vi "CalculateMcsaSpeed[m].vi"(6 "Calculation Cache In":T3 {"speed initial conditions"."zoom FFT settings"."FFT settings"."window" items=["Rectangle"=0, "Hanning"=1, "Hamming"=2, "Blackman-Harris"=3, "Exact Blackman"=4, "Blackman"=5, "Flat Top"=6, "4 Term B-Harris "=7, "7 Term B-Harris"=8, "Low Sidelobe"=9, "Blackman Nuttall"=11, "Triangle"=30, "Bartlett-Hanning"=31, "Bohman"=32, "Parzen"=33, "Welch"=34, "Kaiser"=60, "Dolph-Chebyshev"=61, "Gaussian"=62]; "spectrum initial conditions"."zoom FFT settings"."FFT settings"."window" items=["Rectangle"=0, "Hanning"=1, "Hamming"=2, "Blackman-Harris"=3, "Exact Blackman"=4, "Blackman"=5, "Flat Top"=6, "4 Term B-Harris "=7, "7 Term B-Harris"=8, "Low Sidelobe"=9, "Blackman Nuttall"=11, "Triangle"=30, "Bartlett-Hanning"=31, "Bohman"=32, "Parzen"=33, "Welch"=34, "Kaiser"=60, "Dolph-Chebyshev"=61, "Gaussian"=62]}, 7 "nameplate information":T2, 8 "error in (no error)":errorcluster, 9 "Map":T1, 10 "current waveform":waveform(dbl)[](array[waveform]), 11 "voltage waveform":waveform(dbl)[](array[waveform])) -> (0 "error out":errorcluster, 3 "speed [RPM]":dbl, 4 "Calculation Cache Out":T3 {"speed initial conditions"."zoom FFT settings"."FFT settings"."window" items=["Rectangle"=0, "Hanning"=1, "Hamming"=2, "Blackman-Harris"=3, "Exact Blackman"=4, "Blackman"=5, "Flat Top"=6, "4 Term B-Harris "=7, "7 Term B-Harris"=8, "Low Sidelobe"=9, "Blackman Nuttall"=11, "Triangle"=30, "Bartlett-Hanning"=31, "Bohman"=32, "Parzen"=33, "Welch"=34, "Kaiser"=60, "Dolph-Chebyshev"=61, "Gaussian"=62]; "spectrum initial conditions"."zoom FFT settings"."FFT settings"."window" items=["Rectangle"=0, "Hanning"=1, "Hamming"=2, "Blackman-Harris"=3, "Exact Blackman"=4, "Blackman"=5, "Flat Top"=6, "4 Term B-Harris "=7, "7 Term B-Harris"=8, "Low Sidelobe"=9, "Blackman Nuttall"=11, "Triangle"=30, "Bartlett-Hanning"=31, "Bohman"=32, "Parzen"=33, "Welch"=34, "Kaiser"=60, "Dolph-Chebyshev"=61, "Gaussian"=62]})   [LabVIEW 2017, in "McsaAnalysisFunctions.lvlib"]
uses:
  <vilib>/addons/InsightCM/Utilities/Analysis/MCSA/McsaAnalysisFunctions.lvlib
  <vilib>/addons/InsightCM/Utilities/Analysis/MCSA/controls/McsaCalculationCache.ctl
  <vilib>/addons/Electrical Power/Motor Monitoring/subVIs/ep_Initial Conditions for MCSA Spectra.ctl
  <vilib>/addons/Electrical Power/Motor Monitoring/subVIs/ep_Demodulation Algorithm.ctl
  <vilib>/addons/Electrical Power/Motor Monitoring/subVIs/ep_Zoom FFT Settings.ctl
  <vilib>/addons/Electrical Power/Motor Monitoring/subVIs/ep_Initial Conditions for Speed Estimation.ctl
  <vilib>/addons/PointValueMap/controls/PointMap.ctl
  <vilib>/addons/Electrical Power/Motor Monitoring/subVIs/ep_Spectra Settings.ctl
  <vilib>/addons/Electrical Power/Motor Monitoring/MCSA Spectra (1 Motor with IC).vi
  <vilib>/addons/Electrical Power/Motor Monitoring/NI_EP_Motor Monitoring.lvlib
  <vilib>/addons/PointValueMap/PointValueMap.lvlib
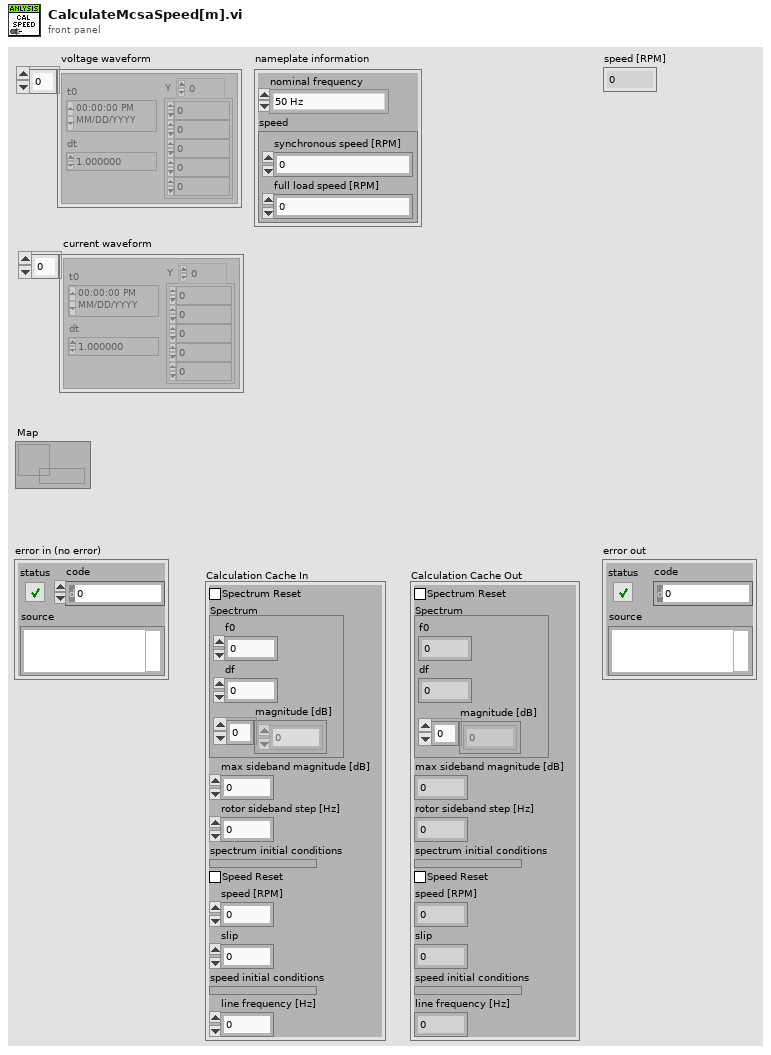
[diagram p1: front panel]
types:
  T1 = typedef "PointValueMap.lvlib/PointMap.ctl" = refnum<data-value>
  T2 = cluster{"nominal frequency":enum16{"50 Hz", "60 Hz"}, "speed":cluster{"synchronous speed [RPM]":dbl, "full load speed [RPM]":dbl}}
  T3 = typedef "McsaAnalysisFunctions.lvlib/McsaCalculationCache.ctl" = cluster{"Spectrum Reset":bool, "Spectrum":cluster{"f0":dbl, "df":dbl, "magnitude [dB]":dbl[]}, "max sideband magnitude [dB]":dbl, "rotor sideband step [Hz]":dbl, "spectrum initial conditions":T4, "Speed Reset":bool, "speed [RPM]":dbl, "slip":dbl, "speed initial conditions":T7, "line frequency [Hz]":dbl}
  T4 = typedef "NI_EP_Motor Monitoring.lvlib/ep_Initial Conditions for MCSA Spectra.ctl" = cluster{"hilbert state":cluster{"delay conditions":dbl[], "filter conditions":dbl[]}, "zoom FFT state":cluster{"phase state":dbl, "zoom FFT state":cluster{"zoom settings state":cluster{"zoom":i32, "stop band attenuation":enum16{"84 dB", "96 dB", "120 dB"}, "alias protect in final transition":bool, "oversampling ratio":dbl}, "SML Decimation Filter (complex input) state":cluster{"decimation settings state":cluster{"M":i32, "stop band attenuation":enum16{"84 dB", "96 dB", "120 dB"}, "alias protect in transition band":bool, "oversampling ratio":dbl}, "counter for garbage samples state":i32, "sml_Parameter Setting for Zoom Factor state":cluster{"filter length * interpolation state":i32, "interpolation state":i32, "comb filter order state":i32, "CFIR par state":cluster{"h":dbl[], "M":i32, "N":i32}, "LFIR par state":cluster{"h":dbl[], "M":i32, "N":i32}, "CIC Stages state":i32}, "aal_CIC (complex input) state":cluster{"aal_cascaded moving average (complex input) state":cluster{"states":cdb[], "circular buffers state":cdb[][], "circular buffer counter state":i32}, "aal_moving average with decimation by order (complex input) state":cluster{"residue result state":cdb, "processed data counter state":i32}}, "sml_Cascaded Decimation Filter (complex input) CFIR state":cluster{"unprocessed data state":cdb[], "final conditions state":cdb[][], "sml_M-1 Decimator with IC (complex input) state":cluster{"coefficients in reverse order state":dbl[], "max index for coefficients state":i32}}, "sml_Cascaded Decimation Filter (complex input) LFIR state":cluster{"unprocessed data state":cdb[], "final conditions state":cdb[][], "sml_M-1 Decimator with IC (complex input) state":cluster{"coefficients in reverse order state":dbl[], "max index for coefficients state":i32}}}, "ma_SML Data Packing (complex input) state":cluster{"array getting packed state":cdb[], "last array processed state":cdb[], "index state":i32, "packing parameters state":cluster{i32, "size":i32}}}, "FFT{X} [Vrms]":cdb[]}, "IIR filter state":cluster{"filter state":dbl[]}, "demodulation settings":cluster{"enable? (F)":bool, "algorithm":T5}, "highpass IIR Filter":cluster{"filter structure":enum32{"IIR 2nd Order", "IIR 4th Order"}, "Reverse Coefficients":dbl[], "Forward Coefficients":dbl[]}, "Hilbert FIR filter":cluster{"coefficients":dbl[], "delay":i32}, "zoom FFT settings":T6}
  T5 = typedef "NI_EP_Motor Monitoring.lvlib/ep_Demodulation Algorithm.ctl" = enum16{"1-phase signal", "3-phase signals"}
  T6 = typedef "NI_EP_Motor Monitoring.lvlib/ep_Zoom FFT Settings.ctl" = cluster{"FFT settings":cluster{"window":u16, "Window Size":i32, "FFT Size":i32, "%overlap":dbl}, "zoom settings":cluster{"zoom":i32, "stop band attenuation":enum16{"84 dB", "96 dB", "120 dB"}, "alias protect in final transition":bool, "oversampling ratio":dbl}, "other settings":cluster{"fmod":dbl, "f0":dbl, "df":dbl, "oidx":i32, "olen":i32}, "iterations":i32, "max block size":i32, "fs":dbl}
  T7 = typedef "NI_EP_Motor Monitoring.lvlib/ep_Initial Conditions for Speed Estimation.ctl" = cluster{"SVAF state":cluster{"space vector amplitude":dbl, "hilbert state":cluster{"delay conditions":dbl[], "filter conditions":dbl[]}}, "zoom FFT state":cluster{"phase state":dbl, "zoom FFT state":cluster{"zoom settings state":cluster{"zoom":i32, "stop band attenuation":enum16{"84 dB", "96 dB", "120 dB"}, "alias protect in final transition":bool, "oversampling ratio":dbl}, "SML Decimation Filter (complex input) state":cluster{"decimation settings state":cluster{"M":i32, "stop band attenuation":enum16{"84 dB", "96 dB", "120 dB"}, "alias protect in transition band":bool, "oversampling ratio":dbl}, "counter for garbage samples state":i32, "sml_Parameter Setting for Zoom Factor state":cluster{"filter length * interpolation state":i32, "interpolation state":i32, "comb filter order state":i32, "CFIR par state":cluster{"h":dbl[], "M":i32, "N":i32}, "LFIR par state":cluster{"h":dbl[], "M":i32, "N":i32}, "CIC Stages state":i32}, "aal_CIC (complex input) state":cluster{"aal_cascaded moving average (complex input) state":cluster{"states":cdb[], "circular buffers state":cdb[][], "circular buffer counter state":i32}, "aal_moving average with decimation by order (complex input) state":cluster{"residue result state":cdb, "processed data counter state":i32}}, "sml_Cascaded Decimation Filter (complex input) CFIR state":cluster{"unprocessed data state":cdb[], "final conditions state":cdb[][], "sml_M-1 Decimator with IC (complex input) state":cluster{"coefficients in reverse order state":dbl[], "max index for coefficients state":i32}}, "sml_Cascaded Decimation Filter (complex input) LFIR state":cluster{"unprocessed data state":cdb[], "final conditions state":cdb[][], "sml_M-1 Decimator with IC (complex input) state":cluster{"coefficients in reverse order state":dbl[], "max index for coefficients state":i32}}}, "ma_SML Data Packing (complex input) state":cluster{"array getting packed state":cdb[], "last array processed state":cdb[], "index state":i32, "packing parameters state":cluster{i32, "size":i32}}}, "FFT{X} [Vrms]":cdb[]}, "speed state":cluster{"speed [RPM]":dbl, "slip":dbl}, "speed estimation settings":cluster{"% overlap":dbl, "algorithm":T5}, "filter information":cluster{"coefficients":dbl[], "order":i32}, "zoom FFT settings":T6, "last valid window":i32, "fund. frequency for averager":dbl[]}
  T8 = typedef "NI_EP_Motor Monitoring.lvlib/ep_Spectra Settings.ctl" = cluster{"number of lines":i32, "% overlap":dbl, "maximum frequency [Hz]":dbl}
  T9 = cluster{"f0":dbl, "df":dbl, "magnitude [dB]":dbl[]}
  T10 = cluster{"spectrum":cluster{"f0":dbl, "df":dbl, "magnitude [dB]":dbl[]}, "demodulated?":bool}
  T11 = cluster{"sideband frequency [Hz]":dbl[], "sideband magnitude [dB]":dbl[]}
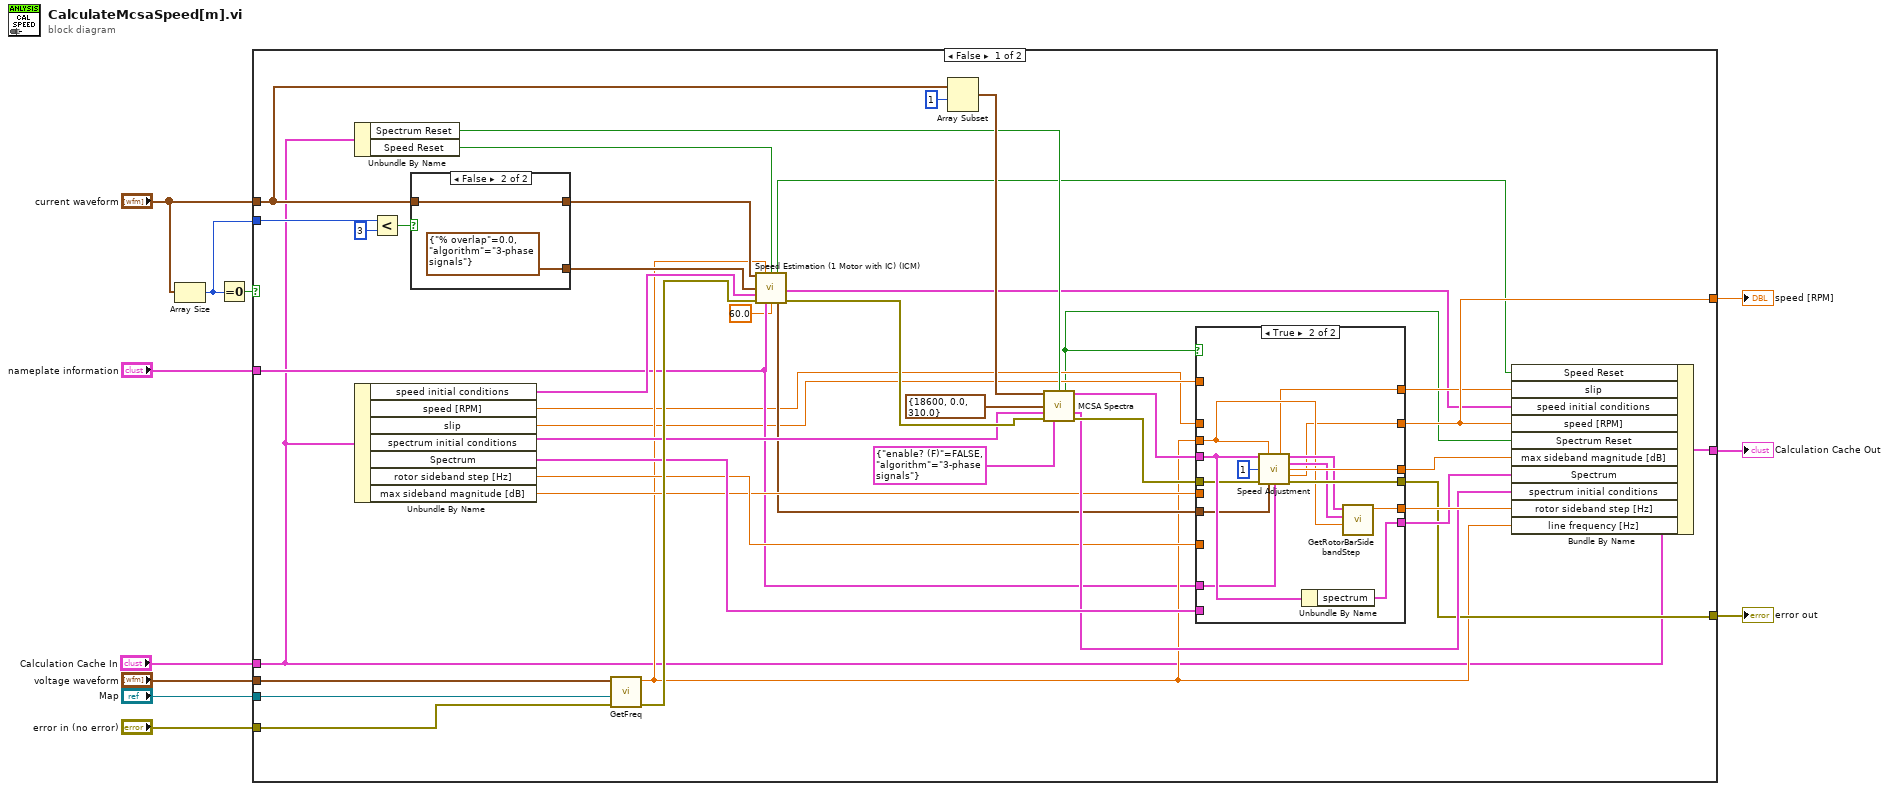
[diagram p0: block diagram]
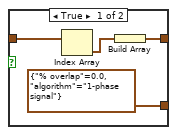
[diagram p3: hidden frame]
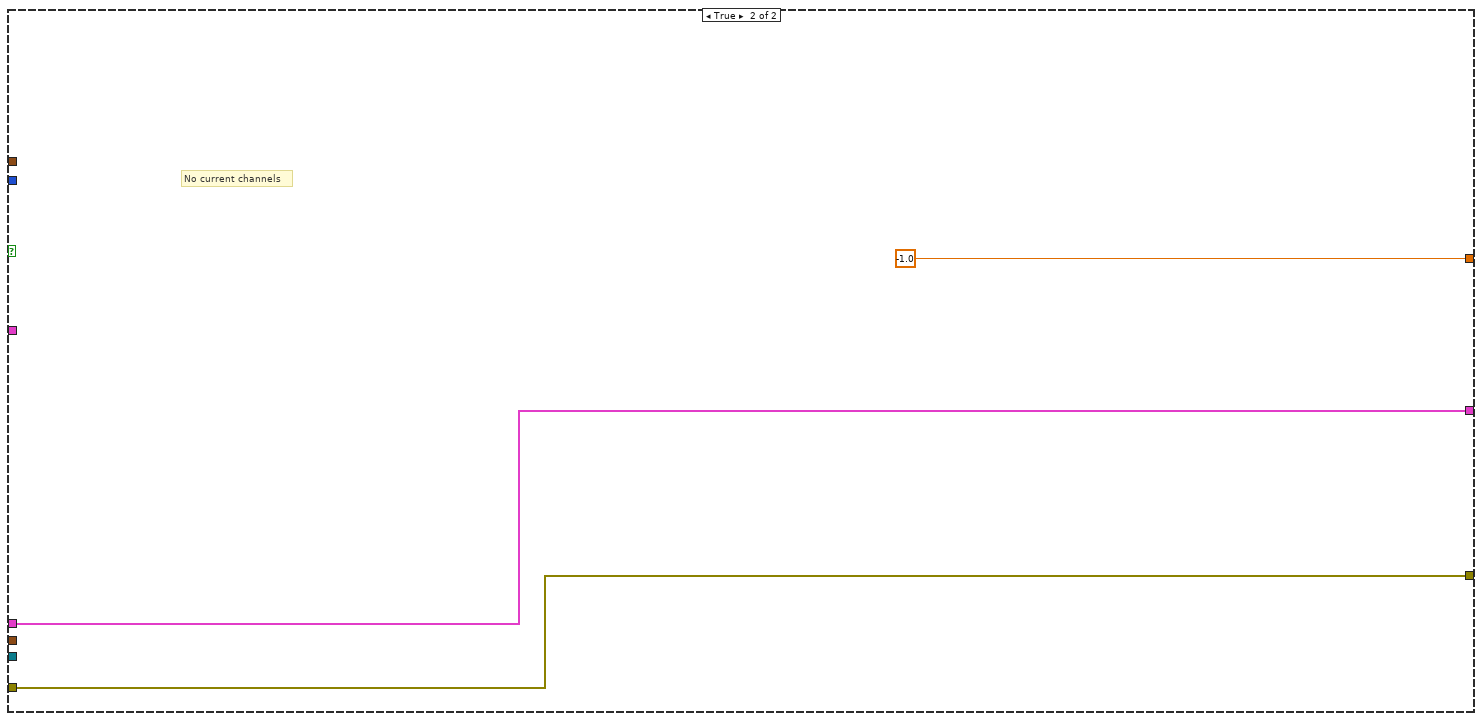
[diagram p4: hidden frame]
diagram:
  n1 = Array Size(array="current waveform") -> (size(s)=w1:i32)
  n2 = Equal To 0?(x=w1) -> (x = 0?=w2:bool)
  n3 = case shown="False" w2 {
    tunnel: "current waveform" -> [w24 _]
    tunnel: [w26 w81] -> w11
    tunnel: [w21 -1.0 ("speed [RPM]")] -> w10
    tunnel: "nameplate information" -> [w20 _]
    tunnel: [w27 w80] -> w8
    tunnel: "error in (no error)" -> [w47 w80]
    tunnel: "Calculation Cache In" -> [w16 w81]
    tunnel: "Map" -> [w46 _]
    tunnel: "voltage waveform" -> [w45 _]
    tunnel: w1 -> [w44 _]
    frame False {
      n4 = Unbundle By Name(w16) -> ("Spectrum Reset"=w36:bool, "Speed Reset"=w51:bool)
      n5 = Unbundle By Name(w16) -> ("speed initial conditions"=w49:T7, "speed [RPM]"=w13:dbl, "slip"=w17:dbl, "spectrum initial conditions"=w37:T4, "Spectrum"=w33:T9, "rotor sideband step [Hz]"=w29:dbl, "max sideband magnitude [dB]"=w28:dbl)
      n6 = Less?(x=w44, y=3) -> (x < y?=w52:bool)
      n7 = case shown="False" w52 {
        tunnel: w24 -> [w77 w79]
        tunnel: [w75 w79] -> w43
        tunnel: [cluster{"% overlap":dbl, "algorithm":T5} {"% overlap"=0.0, "algorithm"=enum."1-phase signal"} ("speed estimation settings") cluster{"% overlap":dbl, "algorithm":T5} {"% overlap"=0.0, "algorithm"=enum."3-phase signals"} ("speed estimation settings")] -> w50
        frame True {
          n8 = Index Array(array=w77) -> (element=w76:waveform(dbl))  [unwired: 1 in]
          n9 = Build Array(w76) -> (w75:waveform(dbl)[])
        }
        frame False {
        }
      }
      n10 = call <vilib>:"GetFreq.vi"("error in (no error)"=w47, "Map"=w46, "waveforms"=w45) -> ("error out"=w48:errorcluster, "frequency"=w23:dbl)  [unwired: 7 in]
      n11 = call <vilib>:"Speed Estimation (1 Motor with IC) (ICM).vi"("waveforms"=w43, "fundamental frequency [Hz]"=w23, "reset? (F)"=w51, "speed estimation settings"=w50, "initial conditions"=w49, "error in (no error)"=w48, "nameplate information"=w20, "window length (60 s)"=60.0) -> ("new data available?"=w14:bool, "final conditions"=w18:T7, "candidate speeds"=w25:cluster{"speed [RPM]":dbl, "slip":dbl}[], "error out"=w38:errorcluster)  [unwired: 2 in, 2 out]
      n12 = Array Subset(array=w24, index=1) -> (w41:waveform(dbl)[])  [unwired: 1 in]
      n13 = call-poly <vilib>:"MCSA Spectra.vi"("waveforms"=w41, "reset? (F)"=w36, "spectrum settings"=T8 {"number of lines"=18600, "% overlap"=0.0, "maximum frequency [Hz]"=310.0}, "initial conditions"=w37, "error in (no error)"=w38, "demodulation settings"=cluster{"enable? (F)":bool, "algorithm":T5} {"enable? (F)"=FALSE, "algorithm"=enum."3-phase signals"}) -> ("new spectrum available?"=w12:bool, "spectrum information"=w35:T10, "final conditions"=w30:T4, "error out"=w34:errorcluster)  [unwired: 6 in]
      n14 = case shown="True" w12 {
        tunnel: w23 -> [_ w65]
        tunnel: w35 -> [_ w72]
        tunnel: [w59 w73] -> w22
        tunnel: w28 -> [w59 _]
        tunnel: [w58 w71] -> w31
        tunnel: w33 -> [w58 _]
        tunnel: w34 -> [w57 w70]
        tunnel: [w57 w69] -> w27
        tunnel: w29 -> [w56 _]
        tunnel: [w56 w67] -> w32
        tunnel: w25 -> [_ w63]
        tunnel: [w55 w64] -> w21
        tunnel: w13 -> [w55 _]
        tunnel: w20 -> [_ w62]
        tunnel: [w54 w61] -> w19
        tunnel: w17 -> [w54 _]
        frame False {
        }
        frame True {
          n15 = call <vilib>:"Speed Adjustment.vi"("spectrum information"=w72, "fundamental frequency [Hz]"=w65, "max sideband order (1)"=u8 1, "error in (no error)"=w70, "candidate speeds"=w63, "nameplate information"=w62) -> ("slip"=w61:dbl, "upper sidebands"=w68:T11, "lower sidebands"=w66:T11, "max sideband magnitude [dB]"=w73:dbl, "speed [RPM]"=w64:dbl, "error out"=w69:errorcluster)  [unwired: 4 in]
          n16 = Unbundle By Name(w72) -> ("spectrum"=w71:T9)
          n17 = call <vilib>:"GetRotorBarSidebandStep.vi"("line frequency [Hz]"=w65, "lower sidebands"=w66, "upper sidebands"=w68) -> ("Rotor Sideband Step [Hz]"=w67:dbl)  [unwired: 8 in]
        }
      }
      n18 = Bundle By Name(cluster=w16, "Speed Reset"=w14, "slip"=w19, "speed initial conditions"=w18, "speed [RPM]"=w21, "Spectrum Reset"=w12, "max sideband magnitude [dB]"=w22, "Spectrum"=w31, "spectrum initial conditions"=w30, "rotor sideband step [Hz]"=w32, "line frequency [Hz]"=w23) -> (w26:T3)
    }
    frame True {
      # "No current channels"
    }
  }
  "speed [RPM]" <- w10
  "Calculation Cache Out" <- w11
  "error out" <- w8
